vi "IMAQdx Close Camera.vi"(8 "error in":errorcluster, 11 "Session In":T1) -> (0 "error out":errorcluster)   [LabVIEW 2020, in "NI_Vision_Acquisition_Software.lvlib"]
doc: "Stops an acquisition in progress, releases resources associated with an acquisition, and closes the specified Camera Session."
uses:
  NI_Vision_Acquisition_Software.lvlib
  IMAQdx.ctl
  niimaqdx.dll
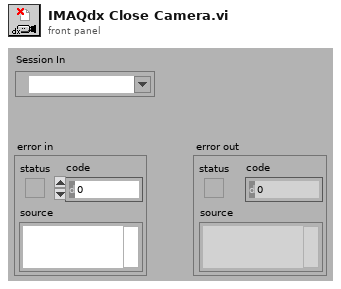
[diagram p1: front panel]
types:
  T1 = typedef "IMAQdx.ctl" = refnum<k21>
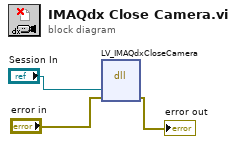
[diagram p0: block diagram]
diagram:
  n1 = dll-call lib="niimaqdx.dll" fn="LV_IMAQdxCloseCamera"("Session In"="Session In", "error in"="error in") -> ("error in"=→"error out":errorcluster)  [unwired: 5 in, 2 out]
